vi "IBM4_Read(V1).vi"(8 "error in":errorcluster, 10 "Channel":enum16{"A2", "A3", "A4", "A5"}(ring), 11 "COM resource in":refnum<visa-resource-name>="COM9") -> (0 "error out":errorcluster, 2 "output":dbl, 3 "COM resource out":refnum<visa-resource-name>)   [LabVIEW 2023, in "IBM4.lvlib"]
doc: "This VI interfaces with the IBM4 to perform a read operation.\n\nThe output will in floating point format (thus, in Volts).\nOnly a single read operation is made with this VI. \n\nAlternate read operations exist covering binary or floating point, single reading, multiple readings, and an average of multiple readings (floating point only)."
uses:
  <instrlib>/IBM4/IBM4.lvlib
panel:
  out "error out 2":errorcluster
  out "read buffer":string
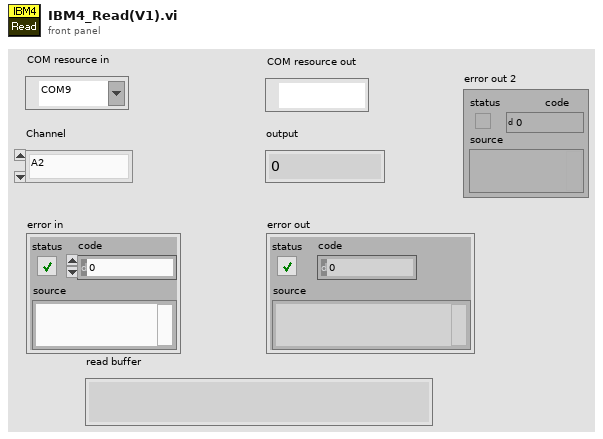
[diagram p1: front panel]
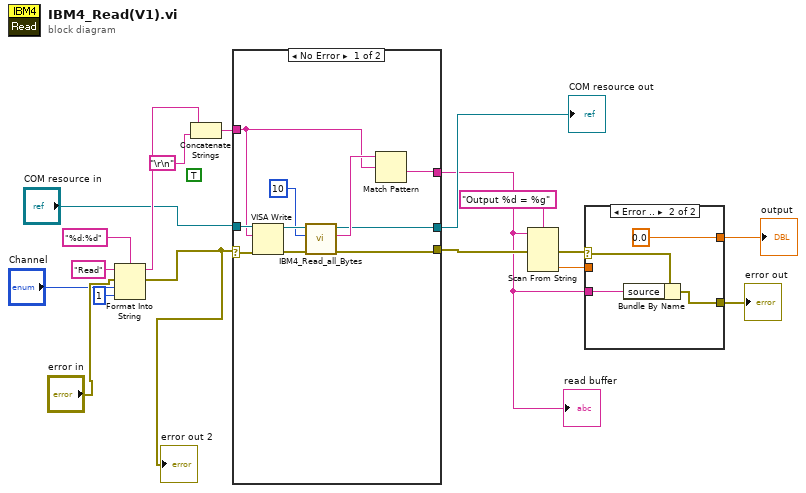
[diagram p0: block diagram]
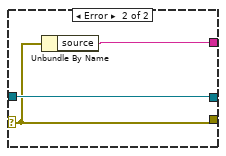
[diagram p3: hidden frame]
diagram:
  (unwired) TRUE ("Enable Termination\nChar (T)")
  n1 = Format Into String(format string="%d:%d", initial string="Read", error in="error in", "Channel", 1 ("input 2")) -> (resulting string=w10:string, error out=w2:errorcluster)
  "error out 2" <- w2
  n2 = Concatenate Strings(w10, "\r\n") -> (w9:string)
  n3 = case shown="No Error" w2 {
    selector: w2 -> [w23 w29]
    tunnel: "COM resource in" -> [w24 w31]
    tunnel: [w21 w29] -> w13
    tunnel: [w19 w30] -> w4
    tunnel: w9 -> [w22 _]
    tunnel: [w20 w31] -> w14
    frame No Error {
      n4 = VISA Write(VISA resource name=w24, write buffer=w22, error in (no error)=w23) -> (VISA resource name out=w27:refnum<visa-resource-name>, error out=w28:errorcluster)  [unwired: 1 out]
      n5 = call <instrlib>:"IBM4_Read_all_Bytes.vi"("error in (no error)"=w28, "milliseconds to wait"=u32 10, "VISA Refnum in"=w27) -> ("error out"=w21:errorcluster, "String"=w26:string, "VISA Refnum out"=w20:refnum<visa-resource-name>)  [unwired: 2 in]
      n6 = Match Pattern(string=w26, regular expression=w22) -> (after substring=w19:string)  [unwired: 1 in, 3 out]
    }
    frame Error {
      n7 = Unbundle By Name(w29) -> ("source"=w30:string)
    }
  }
  "COM resource out" <- w14
  "read buffer" <- w4
  n8 = Scan From String(format string="Output %d = %g", input string=w4, error in=w13) -> (error out=w8:errorcluster, output 2=w7:dbl)  [unwired: 4 in, 2 out]
  n9 = case shown="Error .." w8 {
    selector: w8 -> [w32 w36]
    tunnel: w7 -> [w33 _]
    tunnel: [w33 0.0] -> w6
    tunnel: [w32 w34] -> w5
    tunnel: w4 -> [_ w35]
    frame No Error {
    }
    frame Error {
      n10 = Bundle By Name(cluster=w36, "source"=w35) -> (w34:errorcluster)
    }
  }
  "error out" <- w5
  "output" <- w6
